vi "Config Get Indices.vi"(8 "error in":errorcluster, 9 "Section Name":string, 11 "Config Cluster in":T1) -> (0 "error out":errorcluster, 1 "Value Array":string[](array[string]), 2 "Key Array":string[](array[string]), 3 "Config Cluster out":T1, 5 "Section Index":i32)   [LabVIEW 2017]
uses:
  Config Cluster.ctl
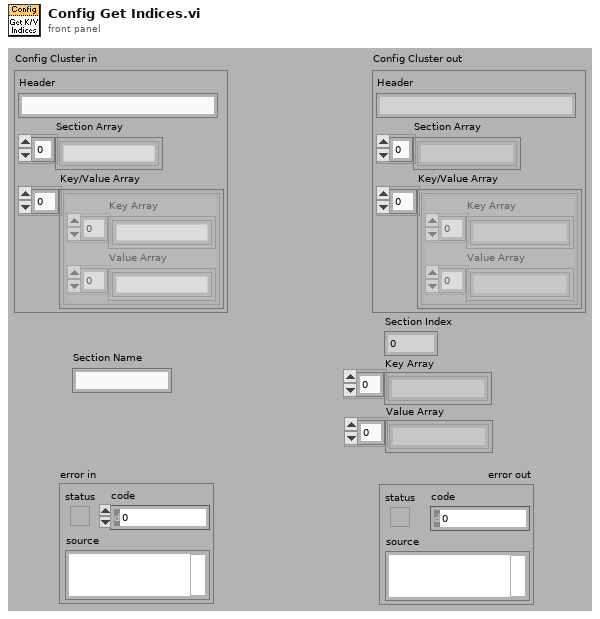
[diagram p1: front panel]
types:
  T1 = typedef "Config Cluster.ctl" = cluster{"Header":string, "Section Array":string[], "Key/Value Array":cluster{"Key Array":string[], "Value Array":string[]}[]}
  T2 = cluster{"Key Array":string[], "Value Array":string[]}[]
  T3 = cluster{"Key Array":string[], "Value Array":string[]}
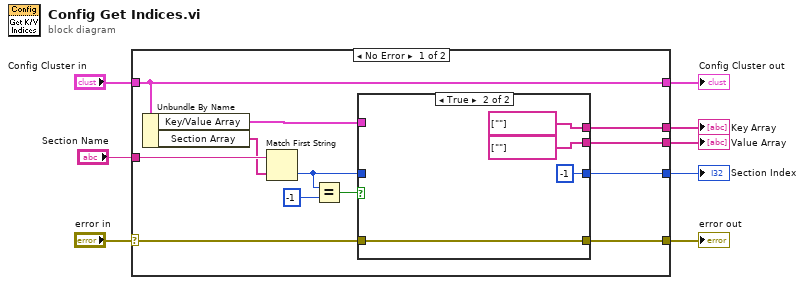
[diagram p0: block diagram]
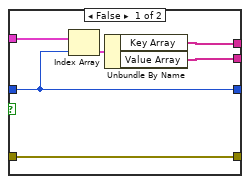
[diagram p2: hidden frame]
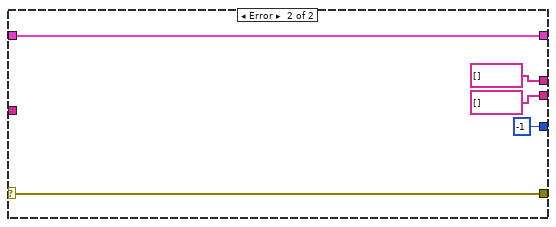
[diagram p3: hidden frame]
diagram:
  n1 = case shown="No Error" "error in" {
    selector: "error in" -> [w16 w34]
    tunnel: [w15 w34] -> w7
    tunnel: "Config Cluster in" -> [w20 w35]
    tunnel: [w20 w35] -> w5
    tunnel: "Section Name" -> [w19 _]
    tunnel: [w12 string[] [] ("Key Array")] -> w3
    tunnel: [w11 -1 ("index")] -> w2
    tunnel: [w9 string[] [] ("Key Array")] -> w1
    frame No Error {
      n2 = Unbundle By Name(w20) -> ("Key/Value Array"=w14:T2, "Section Array"=w10:string[])
      n3 = Match First String(2:w10, 3:w19) -> (0:w13:i32)  [unwired: 1 out]
      n4 = Equal?(x=w13, y=-1) -> (x = y?=w17:bool)
      n5 = case shown="True" w17 {
        tunnel: w16 -> [w26 w27]
        tunnel: [w26 w27] -> w15
        tunnel: w14 -> [w24 _]
        tunnel: w13 -> [w22 _]
        tunnel: [w23 string[] [""] ("Key Array")] -> w12
        tunnel: [w22 -1 ("index")] -> w11
        tunnel: [w21 string[] [""] ("Key Array")] -> w9
        frame False {
          n6 = Index Array(array=w24, index=w22) -> (element=w25:T3)
          n7 = Unbundle By Name(w25) -> ("Key Array"=w23:string[], "Value Array"=w21:string[])
        }
        frame True {
        }
      }
    }
    frame Error {
    }
  }
  "error out" <- w7
  "Config Cluster out" <- w5
  "Key Array" <- w3
  "Section Index" <- w2
  "Value Array" <- w1
